vi "True or false pinout.vi"(0 "VISA Resource Name":refnum<visa-resource-name>, 1 "Input str":string[](array[string]), 2 "State":bool[](array[boolean]), 3 "error in (no error)":errorcluster) -> (6 "VISA Resource Name Out":refnum<visa-resource-name>, 8 "Exir str":string, 9 "error out":errorcluster)   [LabVIEW 2026]
uses:
  <instrlib>/Agilent 34970/Agilent 34970.lvlib
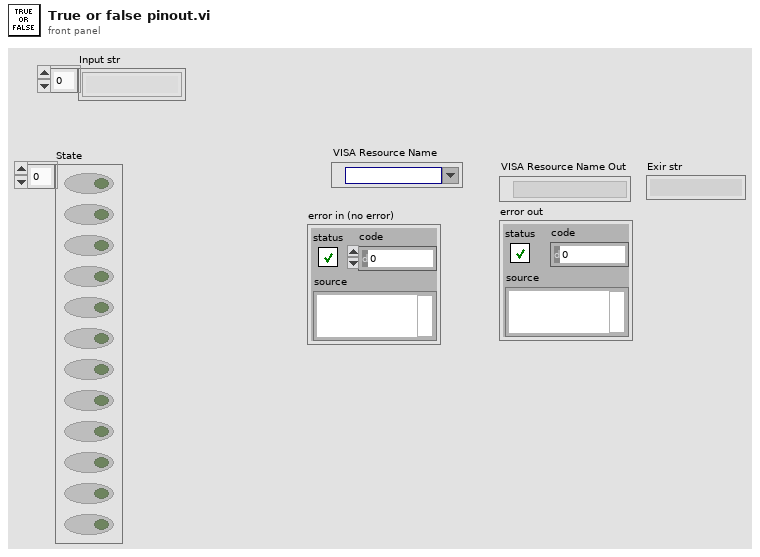
[diagram p1: front panel]
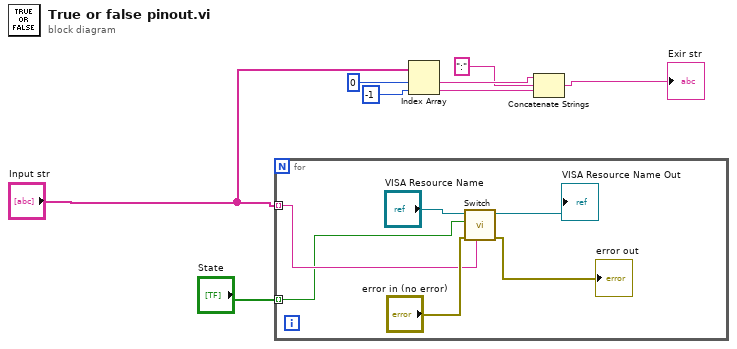
[diagram p0: block diagram]
diagram:
  n1 = for {
    tunnel: "Input str" -> [w12] mode=indexing
    tunnel: "State" -> [w11] mode=indexing
    n2 = call <instrlib>:"Switch.vi"("Channel List(empty)"=w12, "error in (no error)"="error in (no error)", "Open/Close (F:Close)"=w11, "VISA Resource Name"="VISA Resource Name") -> ("error out"=→"error out":errorcluster, "VISA Resource Name Out"=→"VISA Resource Name Out":refnum<visa-resource-name>)  [unwired: 5 in, 1 out]
  }
  n3 = Index Array(array="Input str", index #1=0 ("index"), index #2=-1 ("index")) -> (element #1=w5:string, element #2=w4:string)
  n4 = Concatenate Strings(w5, ":" ("string"), w4) -> (→"Exir str":string)
